vi "AWS-S3-GetProgressEvent.vi"(0 "AWS-S3-API":refnum<class "AWS-S3-API.lvclass">, 11 "error in":errorcluster) -> (4 "AWS-S3-API out":refnum<class "AWS-S3-API.lvclass">, 6 "Object Transfer Events":refnum<event-registration>, 15 "error out":errorcluster)   [LabVIEW 2012, in "AWS-S3-API.lvclass"]
doc: "Note that if you want to catch every single transfer event, call this VI prior to beginning the transfer. This ensures that the Register For Events node is waiting for messages even before events are being sent."
uses:
  AWS-S3-API.lvclass
  AWS-S3-Transfer-Progress.ctl
  AWS-S3-Transfer-Header.ctl
  AWS-S3-Transfer-Completed.ctl
  AWS-S3-API.lvclass/AWS-S3-API.ctl
panel:
  # "Inputs"
  # "Outputs"
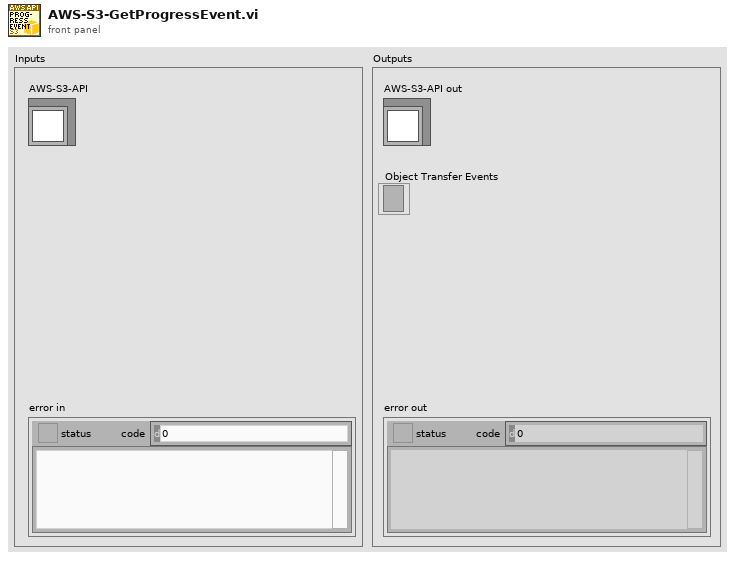
[diagram p1: front panel]
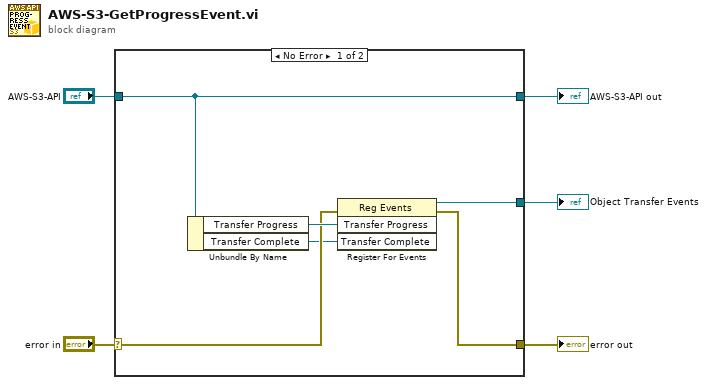
[diagram p0: block diagram]
diagram:
  n1 = case shown="No Error" "error in" {
    selector: "error in" -> [w9 w13]
    tunnel: [w8 w13] -> w5
    tunnel: [w11 w12] -> w3
    tunnel: "AWS-S3-API" -> [w11 w12]
    tunnel: [w7 _] -> w1
    frame No Error {
      n2 = Unbundle By Name(w11) -> ("Transfer Progress"=w10:refnum<user-event>, "Transfer Complete"=w6:refnum<user-event>)
      n3 = register-events(error in=w9, w10, w6) -> (reference out=w7:refnum<event-registration>, error out=w8:errorcluster)  [unwired: 1 in]
    }
    frame Error {
    }
  }
  "error out" <- w5
  "AWS-S3-API out" <- w3
  "Object Transfer Events" <- w1
